vi "Init_Gauge_pump.vi"(3 "Container State":T3, 4 "Previous State":variant, 5 "Previous Version":T2) -> (2 "Current State":T1)   [LabVIEW 2015, in "Gauge_pump.xctl"]
uses:
  Gauge_pump.xctl
  State _Gauge_pump.ctl
  <vilib>/_xctls/Container State.ctl
  <vilib>/_xctls/Version.ctl
  <vilib>/_xctls/XControlSupport.lvlib
panel:
  in  "Default Indicator State":T1
  in  "Default Control State":T1
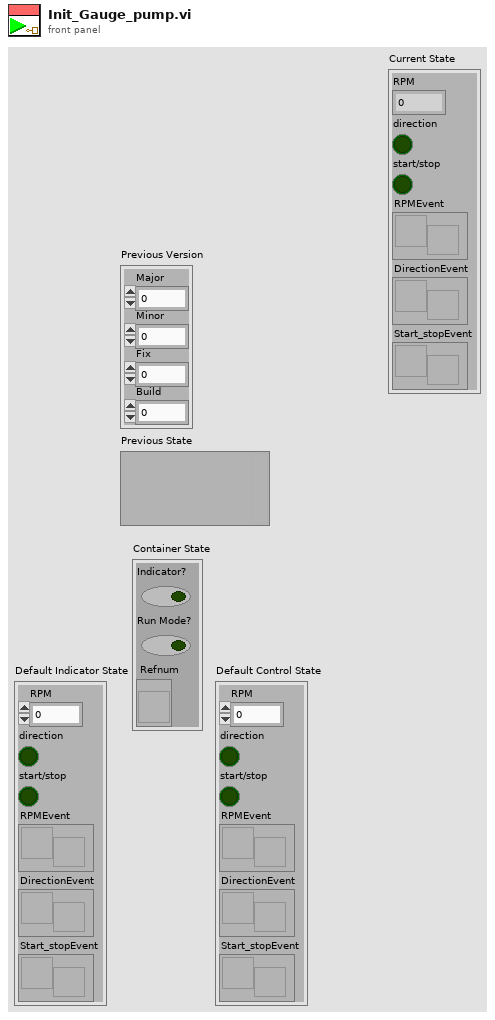
[diagram p1: front panel]
types:
  T1 = typedef "Gauge_pump.xctl/State _Gauge_pump.ctl" = cluster{"RPM":dbl, "direction":bool, "start/stop":bool, "RPMEvent":refnum<user-event>, "DirectionEvent":refnum<user-event>, "Start_stopEvent":refnum<user-event>}
  T2 = typedef "XControlSupport.lvlib/Version.ctl" = cluster{"Major":u16, "Minor":u16, "Fix":u16, "Build":u16}
  T3 = typedef "XControlSupport.lvlib/Container State.ctl" = cluster{"Indicator?":bool, "Run Mode?":bool, " Refnum":refnum<vi>}
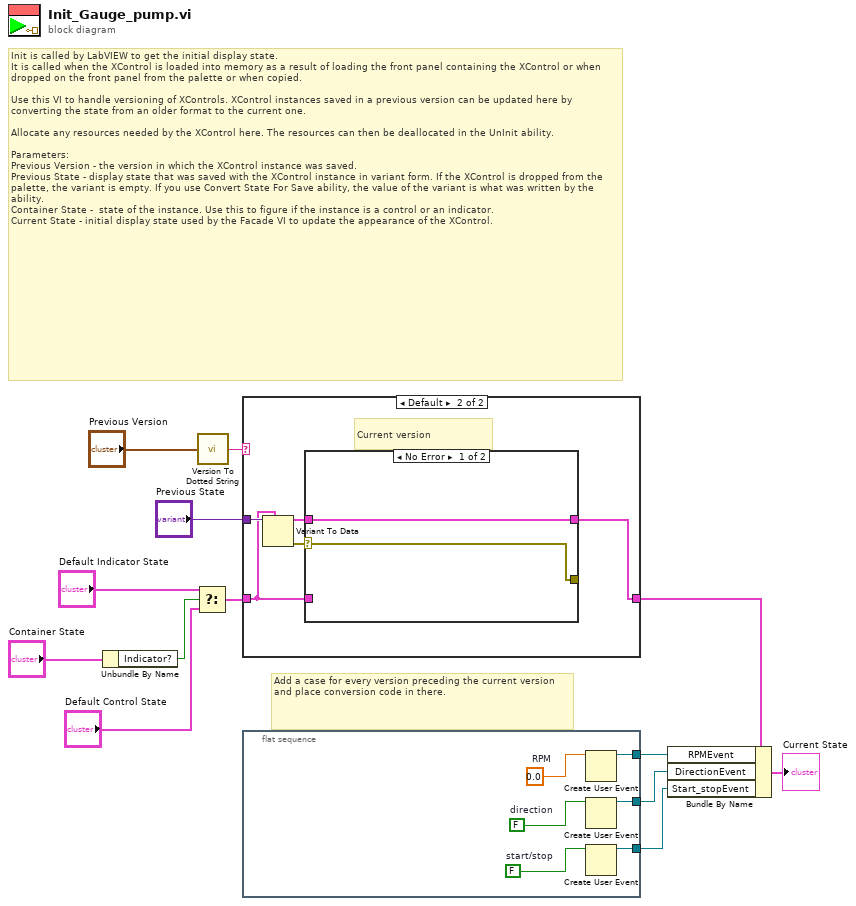
[diagram p0: block diagram]
diagram:
  # "Add a case for every version preceding the current version and place conversion code in there."
  # "Init is called by LabVIEW to get the initial display state.\nIt is called when the XControl is loaded into memory as a result of loading the front panel containing the XControl or when dropped on the front panel from the palette or when copied.\n\nUse this VI to handle versioning of XControls. XControl instances saved in a previous version can be updated here by converting the state from an older format to the current one.\n\nAllocate any resources needed by the XControl here. The resources can then be deallocated in the UnInit ability.\n\nParameters:\nPrevious Version - the version in which the XControl instance was saved.\nPrevious State - display state that was saved with the XControl instance in variant form. If the XControl is dropped from the palette, the variant is empty. If you use Convert State For Save ability, the value of the variant is what was written by the ability. \nContainer State -  state of the instance. Use this to figure if the instance is a control or an indicator.\nCurrent State - initial display state used by the Facade VI to update the appearance of the XControl."
  n1 = Unbundle By Name("Container State") -> ("Indicator?"=w9:bool)
  n2 = Select(t="Default Indicator State", s=w9, f="Default Control State") -> (s? t:f=w8:T1)
  n3 = call <vilib>:"Version To Dotted String.vi"("Version"="Previous Version") -> ("String Version"=w6:string)
  n4 = case shown="Default" w6 {
    tunnel: "Previous State" -> [_ w19]
    tunnel: [w14 w15] -> w5
    tunnel: w8 -> [w14 w16]
    frame "0.0.0.0" {
      # "Just created, use default state"
    }
    frame Default {
      # "Current version"
      n5 = Variant To Data(type=w16, Variant=w19) -> (data=w17:T1, error out=w18:errorcluster)  [unwired: 1 in]
      n6 = case shown="No Error" w18 {
        selector: w18 -> [w21 w22]
        tunnel: w17 -> [w20 _]
        tunnel: [w20 w23] -> w15
        tunnel: w16 -> [_ w23]
        tunnel: [w21 w22] -> _
        frame No Error {
        }
        frame Error {
          # "Error converting previously \nsaved state. Use default instead."
        }
      }
    }
  }
  n7 = flat-sequence {
    tunnel: [w26] -> w3
    tunnel: [w25] -> w2
    tunnel: [w24] -> w1
    frame #0 {
      w27 = FALSE  # direction
      w28 = FALSE  # start/stop
      w29 = 0.0  # RPM
      n8 = Create User Event(user event datatype=w29) -> (user event=w26:refnum<user-event>)  [unwired: 1 in, 1 out]
      n9 = Create User Event(user event datatype=w27) -> (user event=w25:refnum<user-event>)  [unwired: 1 in, 1 out]
      n10 = Create User Event(user event datatype=w28) -> (user event=w24:refnum<user-event>)  [unwired: 1 in, 1 out]
    }
  }
  n11 = Bundle By Name(cluster=w5, "RPMEvent"=w3, "DirectionEvent"=w2, "Start_stopEvent"=w1) -> (→"Current State":T1)
